vi "GDSLvIcon_ManageIconFolderDialog.vi"(8 "error in (no error)":errorcluster) -> (0 "error out":errorcluster, 3 "Cancelled":bool)   [LabVIEW 2020]
panel:
  in  "_Cancel":bool
  in  "_OK":bool
  in  "_IconFolders":path[](array[path]) caption="Icon Folders"
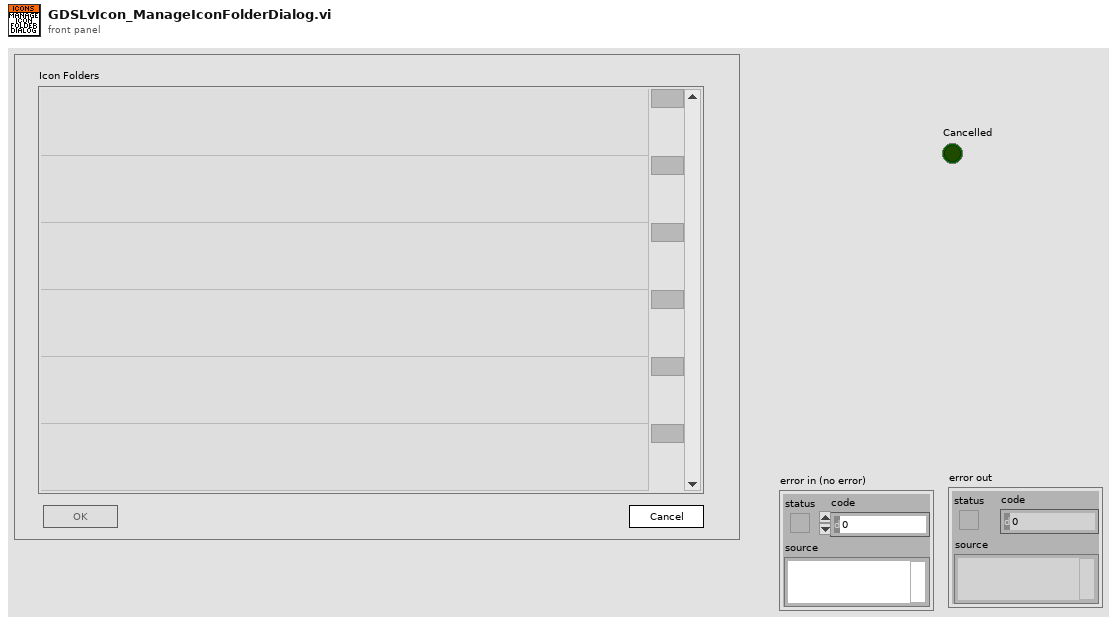
[diagram p1: front panel]
types:
  T1 = cluster{"Counter":i32, "Text":string, "Cancelled":bool}
  T2 = enum8{"Enabled", "Disabled", "Disabled and Grayed Out"}
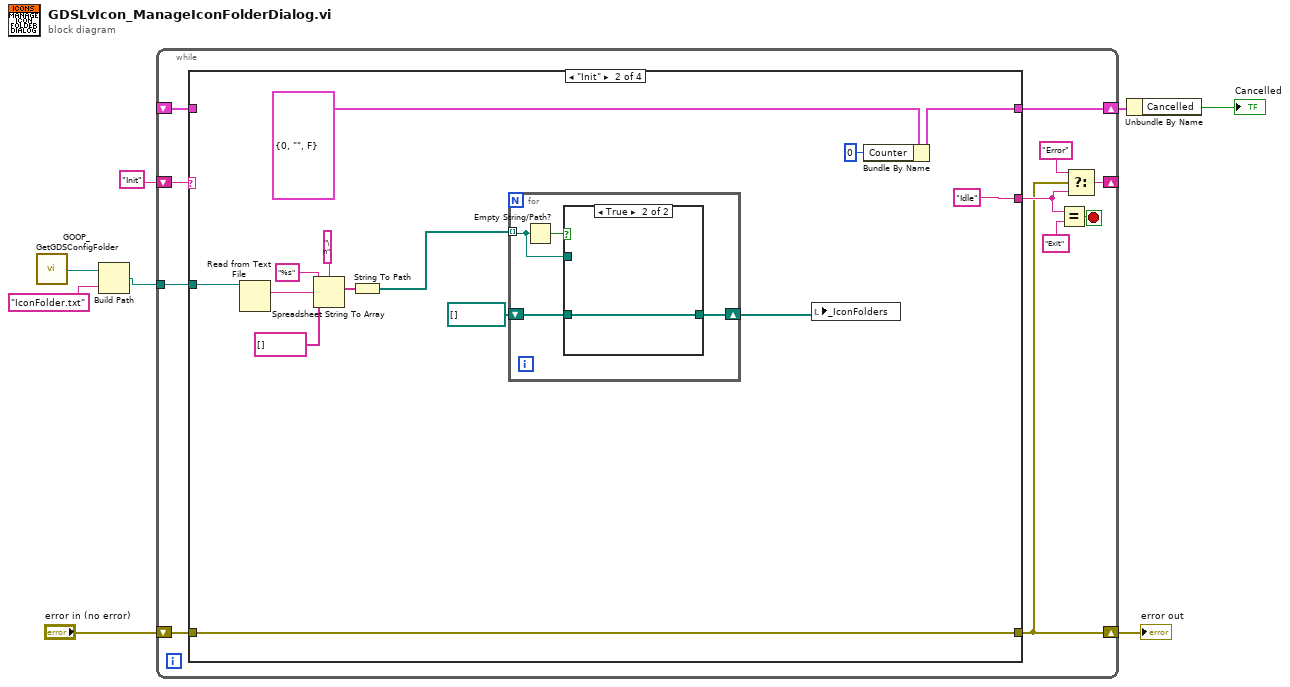
[diagram p0: block diagram]
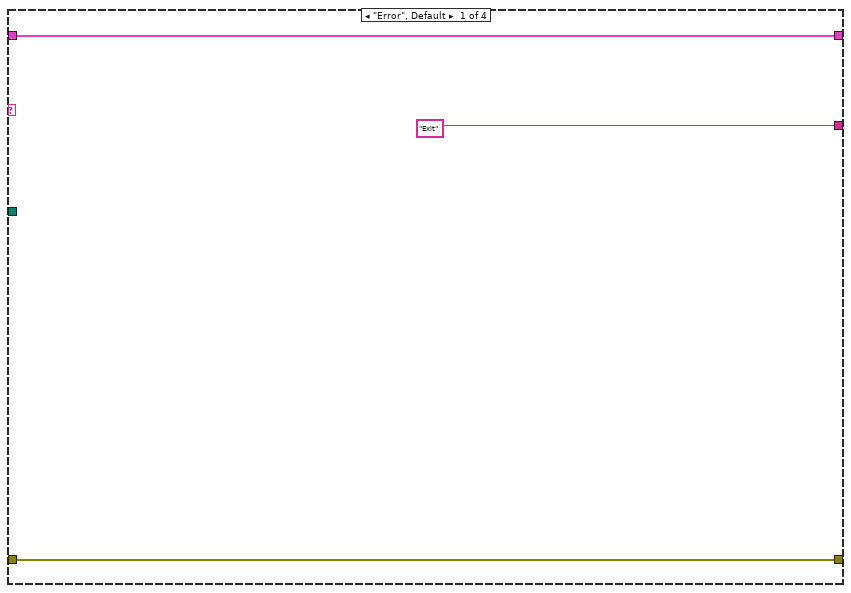
[diagram p2: hidden frame]
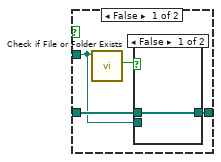
[diagram p3: hidden frame]
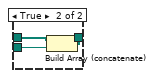
[diagram p4: hidden frame]
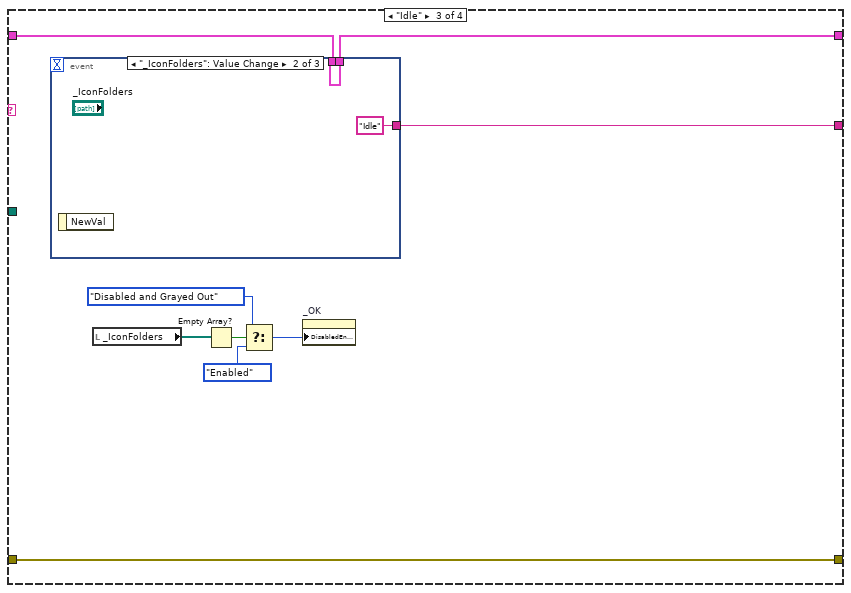
[diagram p5: hidden frame]
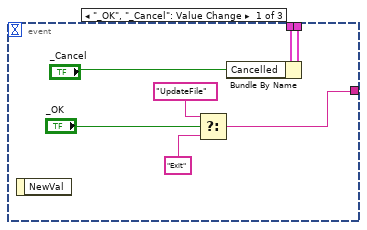
[diagram p6: hidden frame]
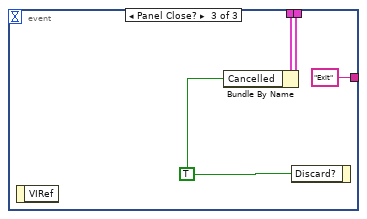
[diagram p7: hidden frame]
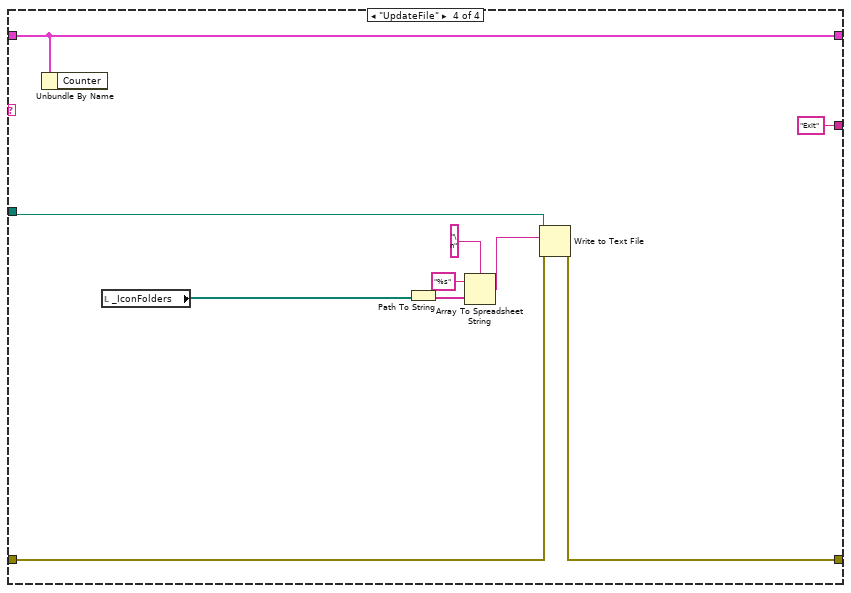
[diagram p8: hidden frame]
diagram:
  n1 = call <resource>:"GOOP_GetGDSConfigFolder.vi"() -> ("GDSFolderPath"=w3:path)
  n2 = Build Path(base path=w3, name or relative path="IconFolder.txt") -> (appended path=w2:path)
  n3 = while {
    shift-right: [w12] -> w5
    shift-left: "error in (no error)" -> [w19]
    shift-right: [w17] -> _
    shift-left: "Init" -> [w18]
    shift-right: [w11] -> w8
    shift-left: _ -> [w10]
    tunnel: w2 -> [w9]
    stop <- w16 stop-if-true
    n4 = case shown="\"Init\"" w18 {
      tunnel: w19 -> [w22 w26 w55 w73]
      tunnel: [w22 w26 w55 w72] -> w12
      tunnel: ["Exit" "Idle" w56 "Exit"] -> w13
      tunnel: [w20 w34 w57 w80] -> w11
      tunnel: w10 -> [w20 _ w58 w80]
      tunnel: w9 -> [_ w27 _ w74]
      frame "Error", Default {
      }
      frame "Init" {
        n5 = Read from Text File(file (use dialog)=w27) -> (text=w32:string)  [unwired: 3 in, 3 out]
        n6 = Spreadsheet String To Array(delimiter (Tab)="\n", format string="%s", spreadsheet string=w32, array type (2D Dbl)=string[] []) -> (array=w28:string[])
        n7 = String To Path(string=w28) -> (path=w24:path[])
        n8 = for {
          tunnel: w24 -> [w39] mode=indexing
          shift-right: [w37] -> w23
          shift-left: path[] [] -> [w38]
          n9 = Empty String/Path?(string/path=w39) -> (empty?=w40:bool)
          n10 = case shown="True" w40 {
            tunnel: w39 -> [w41 _]
            tunnel: w38 -> [w44 w49]
            tunnel: [w43 w49] -> w37
            frame False {
              n11 = call <vilib>:"Check if File or Folder Exists.vi"("path"=w41) -> ("file or folder exists?"=w42:bool)  [unwired: 8 in, 2 out]
              n12 = case shown="False" w42 {
                tunnel: w44 -> [w45 w48]
                tunnel: [w45 w47] -> w43
                tunnel: w41 -> [_ w46]
                frame False {
                }
                frame True {
                  n13 = Build Array (concatenate)(w48, w46) -> (w47:path[])
                }
              }
            }
            frame True {
            }
          }
        }
        n14 = local write "_IconFolders"(w23) -> ()
        n15 = Bundle By Name(cluster=T1 {"Counter"=0, "Text"="", "Cancelled"=FALSE}, "Counter"=0) -> (w34:T1)
      }
      frame "Idle" {
        n16 = event shown="[1] \"_IconFolders\": Value Change" {
          selector: _ -> [_ _ _]
          dyn-events: _ -> [_ _ _]
          timeout: _ -> [_ _ _]
          tunnel: w58 -> [w65 w66 w70]
          tunnel: [w64 w66 w69] -> w57
          tunnel: [w61 "Idle" "Exit"] -> w56
          event "_OK", "_Cancel": Value Change {
            n17 = event-data() -> ()  [unwired: 1 in, 1 out]
            n18 = Select(t="UpdateFile", s="_OK", f="Exit") -> (s? t:f=w61:string)
            n19 = Bundle By Name(cluster=w65, "Cancelled"="_Cancel") -> (w64:T1)
          }
          event "_IconFolders": Value Change {
            n20 = event-data() -> ()  [unwired: 1 in, 1 out]
          }
          event Panel Close? {
            w68 = TRUE ("Discard?")
            n21 = event-data() -> ()  [unwired: 1 in, 1 out]
            n22 = Bundle By Name(cluster=w70, "Cancelled"=w68) -> (w69:T1)
            n23 = event-data("Discard?"=w68) -> ()  [unwired: 1 in, 1 out]
          }
        }
        n24 = local read "_IconFolders"() -> (w54:path[])
        n25 = Empty Array?(array=w54) -> (empty?=w53:bool)
        n26 = Select(t=T2."Disabled and Grayed Out", s=w53, f=T2."Enabled" ("Disabled")) -> (s? t:f=w51:T2)
        n27 = property on="_OK" class="Bool"("DisabledEnum"=w51) -> ()  [unwired: 2 in, 2 out]
      }
      frame "UpdateFile" {
        n28 = Unbundle By Name(w80) -> ()  [unwired: 1 out]
        n29 = local read "_IconFolders"() -> (w79:path[])
        n30 = Path To String(path=w79) -> (string=w78:string[])
        n31 = Array To Spreadsheet String(delimiter (Tab)="\n", array=w78, 3:"%s" ("format string")) -> (spreadsheet string=w75:string)
        n32 = Write to Text File(file (use dialog)=w74, text=w75, error in=w73) -> (error out=w72:errorcluster)  [unwired: 1 in, 2 out]
      }
    }
    n33 = Equal?(x=w13, y="Exit") -> (x = y?=w16:bool)
    n34 = Select(t="Error", s=w12, f=w13) -> (s? t:f=w17:string)
  }
  "error out" <- w5
  n35 = Unbundle By Name(w8) -> ("Cancelled"=→"Cancelled":bool)
